vi "Messaging EnQ Multiple.vi"(5 "[Commands]":string[](array[string]), 6 "@Front?":bool, 7 "[Data]":variant[](array[variant]), 8 "error in (no error)":errorcluster) -> (0 "error out":errorcluster)   [LabVIEW 2019, in "GUI.lvlib"]
doc: "Enqueue multiple <b>[Commands]</b> with variant <b>[Data]</b>. Optionally choose if you want the element <b>@Front</b> of the Q."
uses:
  GUI.lvlib
  Private Controls/Messaging Data.ctl
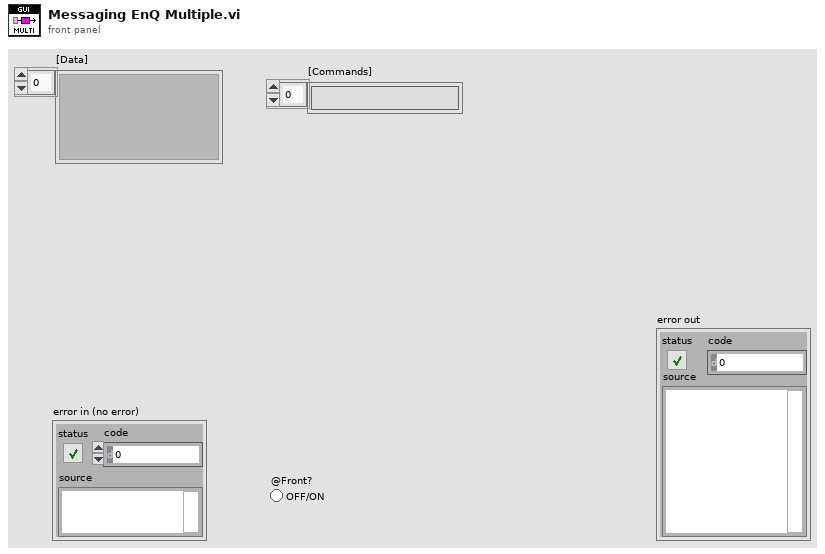
[diagram p1: front panel]
types:
  T1 = typedef "GUI.lvlib/Messaging Data.ctl" = cluster{"Command":string, "Data":variant}
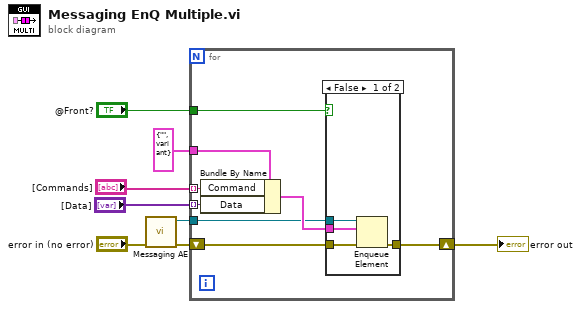
[diagram p0: block diagram]
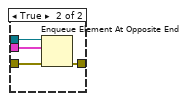
[diagram p2: hidden frame]
diagram:
  n1 = call "Messaging AE.vi"("Error In"="error in (no error)") -> ("Error Out"=w5:errorcluster, "queue out"=w4:refnum<queue>)  [unwired: 9 in]
  n2 = for {
    tunnel: T1 {"Command"="", "Data"=variant} ("Message Data") -> [w14]
    tunnel: "@Front?" -> [w13]
    tunnel: w4 -> [w11]
    tunnel: "[Data]" -> [w10] mode=indexing
    tunnel: "[Commands]" -> [w9] mode=indexing
    shift-right: [w16] -> w8
    shift-left: w5 -> [w12]
    n3 = Bundle By Name(cluster=w14, "Command"=w9, "Data"=w10) -> (w15:T1)
    n4 = case shown="False" w13 {
      tunnel: w15 -> [w20 w24]
      tunnel: w11 -> [w19 w23]
      tunnel: [w18 w22] -> w16
      tunnel: w12 -> [w17 w21]
      frame False {
        n5 = Enqueue Element(queue=w19, element=w20, error in (no error)=w17) -> (error out=w18:errorcluster)  [unwired: 1 in, 2 out]
      }
      frame True {
        n6 = Enqueue Element At Opposite End(queue=w23, element=w24, error in (no error)=w21) -> (error out=w22:errorcluster)  [unwired: 1 in, 2 out]
      }
    }
  }
  "error out" <- w8
